vi "VisionDataNetwork.vi"() -> ()   [LabVIEW 2011]
panel:
  in  "VisionDataOverNetwork":T1
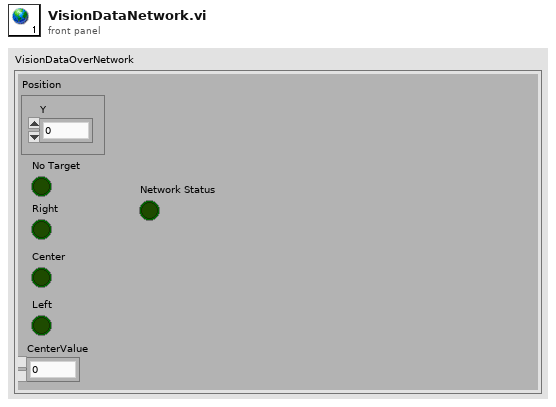
[diagram p1: front panel]
types:
  T1 = cluster{"Position":cluster{"Y":dbl}, "No Target":bool, "Right":bool, "Center":bool, "Left":bool, "CenterValue":dbl, "Network Status":bool}
diagram:
